vi "Script Find current Error Codes.vi"(8 "error in":errorcluster, 11 "Selection Owning Folder":path) -> (0 "error out":errorcluster, 1 "All Error VIS":path[](array[path]), 2 "Error and Descriptions Table":string[][](array[string]))   [LabVIEW 2020, in "ConstantErrorsMaker.lvlib"]
uses:
  ConstantErrorsMaker.lvlib
  <vilib>/Utility/traverseref.llb/TRef TravTarget.ctl
  c460e84f-7e8e-40e4-832a-a8e949bfd169.vi
  <vilib>/Comparison/Less/Less Functor/Less Functor.lvclass
  <vilib>/Utility/traverseref.llb/VI Scripting - Traverse.lvlib
  Error Info--cluster.ctl
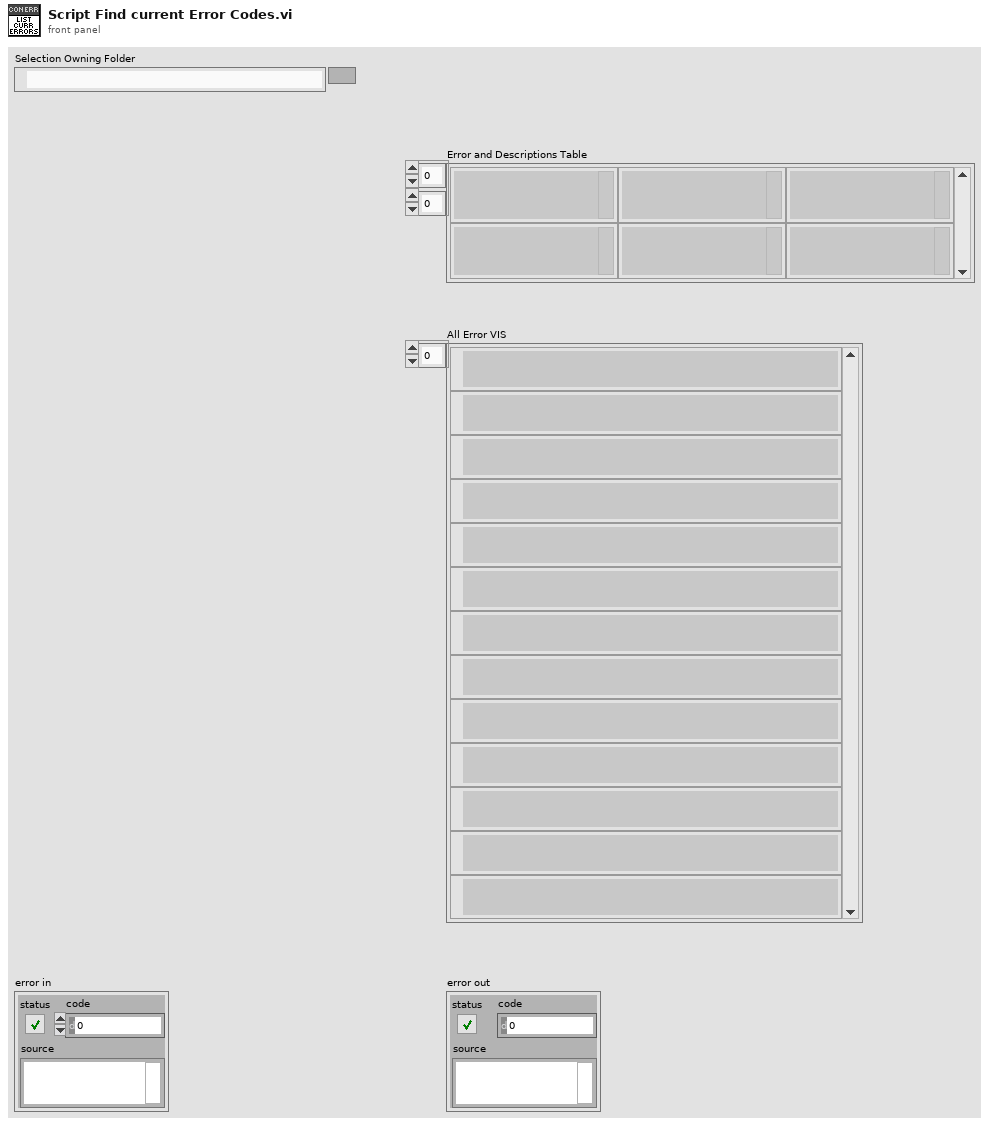
[diagram p1: front panel]
types:
  T1 = typedef "ConstantErrorsMaker.lvlib/Error Info--cluster.ctl" = cluster{"Error Code":i32, "Error Description":string, "Parent":string, "Error Path":path}
  T2 = typedef "TRef TravTarget.ctl" = enum16{"FP", "BD", "Other"}
  T3 = cluster{"Clipped Error Description":string, "Full Error Description":string, "code":i32, "Family":string, "Custom Description":string, "Is Error":bool, "Types":variant[], "Include Call Chain?":bool, "Error Text Visible":bool}
  T4 = cluster{"Library Version":cluster{"Major":u16, "Minor":u16, "Fix":u16, "Build":u16}, "State":variant}
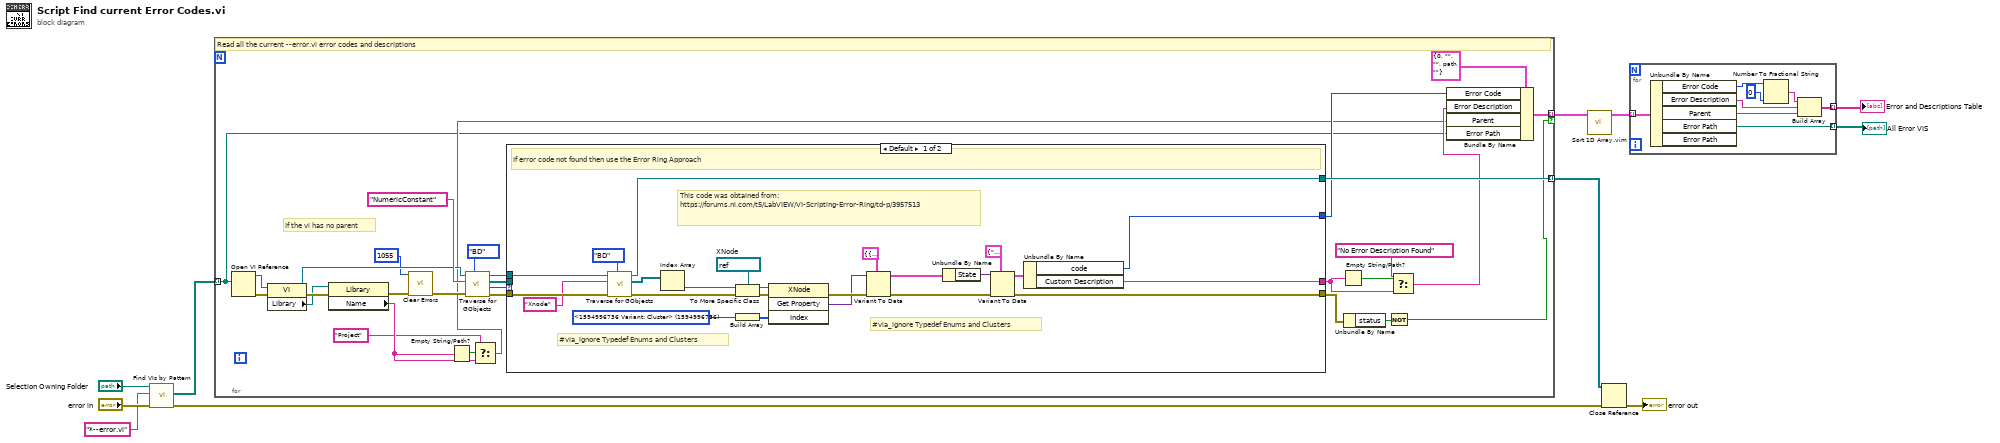
[diagram p0: block diagram]
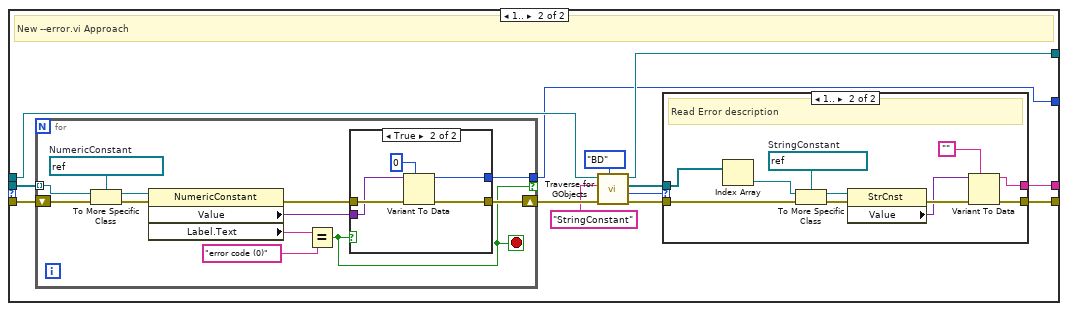
[diagram p2: hidden frame]
diagram:
  n1 = call "Find VIs by Pattern.vi"("error in"="error in", "pattern"="*--error.vi", "Selction Owning Folder"="Selection Owning Folder") -> ("error out"=w10:errorcluster, "All Files in Dir"=w7:path[])  [unwired: 7 in]
  n2 = for {
    tunnel: w7 -> [w12] mode=indexing
    tunnel: [w30] -> w6 mode=indexing
    tunnel: [w17] -> w4 mode=indexing if=w16
    # "If the vi has no parent"
    # "Read all the current --error.vi error codes and descriptions"
    n3 = Open VI Reference(vi path=w12) -> (vi reference=w25:refnum<vi>, error out=w40:errorcluster)  [unwired: 5 in]
    n4 = property class="VI"(reference=w25, error in=w40) -> (reference out=w24:refnum<vi>, error out=w38:errorcluster, "Library"=w23:refnum<vi>)
    n5 = property class="Library"(reference=w23, error in=w38) -> (error out=w37:errorcluster, "Name"=w21:string)  [unwired: 1 out]
    n6 = call <vilib>:"Clear Errors.vi"("error in (no error)"=w37, "specific error code to clear (0: all)"=1055) -> ("error out"=w36:errorcluster)  [unwired: 4 in, 1 out]
    n7 = Empty String/Path?(string/path=w21) -> (empty?=w22:bool)
    n8 = call <vilib>:"Traverse for GObjects.vi"("Traverse Target"=TRef_TravTarget."BD", "error in (no error)"=w36, "Class Name"="NumericConstant", "VI Refnum"=w24) -> ("error out"=w41:errorcluster, "# of Refs"=w32:i32, "References"=w34:refnum<vi>[], "dup VI Refnum"=w31:refnum<vi>)  [unwired: 4 in]
    n9 = Select(t="Project", s=w22, f=w21) -> (s? t:f=w13:string)
    n10 = case shown="Default" w32 {
      tunnel: [w44 w66] -> w15
      tunnel: [w62 w77] -> w39
      tunnel: w41 -> [w65 w76]
      tunnel: w34 -> [_ w74]
      tunnel: w31 -> [w57 w69]
      tunnel: [w43 w68] -> w27
      tunnel: [w42 w67] -> w30
      frame Default {
        w53 = u32 1594996736 items=["<1594996736 Variant: Cluster>"=1594996736, "<1594996767 Diagram RefNum>"=1594996737, "<1594996738 ProjectItem Refnum>"=1594996738, "<1594996739 Boolean>"=1594996739, "<1594996740 Boolean>"=1594996740, "<1594996741 Boolean>"=1594996741, "<1594996742 String: .html file name>"=1594996742, "<1594996743 Help Path>"=1594996743, "<1594996744 String: Tip Strip>"=1594996744, "<1594996745 Boolean>"=1594996745, "<104204298 Boolean>"=104204298, "AutoSize To Fit Contents?"=104204288, "Basic Object Flags"=103983116, "Bounds"=103983107, "Bounds:Area Height"=103983109, "Bounds:Area Width"=103983108, "Breakpoint Status"=104173580, "Clump Num"=104173572, "Content Rect"=104204293, "Description"=104173570, "Diagrams[]"=104204291, "Fire Count"=104173574, "Fix Contents"=104204297, "Frame Size"=104204290, "Icon"=104173576, "Is Asynchronous"=104173575, "Is Break Point Set"=104173571, "Is Run At Any Loop"=104173578, "Is Wizard Locked"=103983117, "Label"=104173569, "Master Bounds Rect"=103983115, "Position"=103983104, "Position:Left"=103983105, "Position:Top"=103983106, "Resize Info:Can Resize Horizontally"=103983119, "Resize Info:Can Resize Vertically"=103983120, "Resize Info:Include In Resize"=103983122, "Resize Info:Name in Resize Dialog"=103983121, "Selected"=103983113, "Shared Clones:Automatic Allocation Strategy Enabled"=104204295, "Shared Clones:Pre-Allocate"=104204296, "Short Count"=104173573, "Style"=104173577, "Target Syntax Checking"=104204292, "Terminals[]"=104173568, "Total Bounds Rect"=103983114, "Tunnels[]"=104204289, "UID"=103983123]
        w56 = refnum<vi> refnum  # XNode
        # "#via_ignore Typedef Enums and Clusters"
        # "#via_ignore Typedef Enums and Clusters"
        # "This code was obtained from:\nhttps://forums.ni.com/t5/LabVIEW/VI-Scripting-Error-Ring/td-p/3957513"
        # "If error code not found then use the Error Ring Approach"
        n11 = call <vilib>:"Traverse for GObjects.vi"("Traverse Target"=TRef_TravTarget."BD", "error in (no error)"=w65, "Class Name"="Xnode", "VI Refnum"=w57) -> ("error out"=w64:errorcluster, "References"=w55:refnum<vi>[], "dup VI Refnum"=w42:refnum<vi>)  [unwired: 4 in, 1 out]
        n12 = Index Array(array=w55) -> (element=w54:refnum<vi>)  [unwired: 1 in]
        n13 = To More Specific Class(target class=w56, reference=w54, error in=w64) -> (specific class reference=w52:refnum<vi>, error out=w63:errorcluster)
        n14 = Build Array(w53) -> (w51:u32[])
        n15 = invoke class="XNode" method="Get Property"(reference=w52, error in=w63, "Index"=w51) -> (error out=w61:errorcluster, "GetProperty"=w46:variant)  [unwired: 1 in, 2 out]
        n16 = Variant To Data(error in=w61, type=T4 {"Library Version"={"Major"=0, "Minor"=0, "Fix"=0, "Build"=0}, "State"=variant} ("output cluster"), Variant=w46) -> (data=w50:T4, error out=w60:errorcluster)
        n17 = Unbundle By Name(w50) -> ("State"=w48:variant)
        n18 = Variant To Data(error in=w60, type=T3 {"Clipped Error Description"="", "Full Error Description"="", "code"=0, "Family"="", "Custom Description"="", "Is Error"=TRUE, "Types"=[], "Include Call Chain?"=TRUE, "Error Text Visible"=TRUE} ("State"), Variant=w48) -> (data=w45:T3, error out=w62:errorcluster)
        n19 = Unbundle By Name(w45) -> ("code"=w44:i32, "Custom Description"=w43:string)
      }
      frame 1.. {
        # "New --error.vi Approach"
        n20 = for {
          tunnel: w74 -> [w86] mode=indexing
          tunnel: [w80] -> w66 if=w79
          shift-right: [w87] -> w75
          shift-left: w76 -> [w90]
          stop <- w79 stop-if-true
          w85 = refnum<vi> refnum  # NumericConstant
          n21 = To More Specific Class(target class=w85, reference=w86, error in=w90) -> (specific class reference=w84:refnum<vi>, error out=w89:errorcluster)
          n22 = property class="NumericConstant"(reference=w84, error in=w89) -> (error out=w88:errorcluster, "Value"=w81:variant, "Label.Text"=w83:string)  [unwired: 1 out]
          n23 = Equal?(x=w83, y="error code (0)") -> (x = y?=w79:bool)
          n24 = case shown="True" w79 {
            tunnel: w81 -> [_ w93]
            tunnel: w88 -> [w91 w96]
            tunnel: [w91 w95] -> w87
            tunnel: [_ w92] -> w80
            frame False {
            }
            frame True {
              n25 = Variant To Data(error in=w96, type=0, Variant=w93) -> (data=w92:i32, error out=w95:errorcluster)
            }
          }
        }
        n26 = call <vilib>:"Traverse for GObjects.vi"("Traverse Target"=TRef_TravTarget."BD", "error in (no error)"=w75, "Class Name"="StringConstant", "VI Refnum"=w69) -> ("error out"=w78:errorcluster, "# of Refs"=w70:i32, "References"=w73:refnum<vi>[], "dup VI Refnum"=w67:refnum<vi>)  [unwired: 4 in]
        n27 = case shown="1.." w70 {
          tunnel: [_ w104] -> w68
          tunnel: [w97 w108] -> w77
          tunnel: w78 -> [w97 w107]
          tunnel: w73 -> [_ w99]
          frame Default {
          }
          frame 1.. {
            w103 = refnum<vi> refnum  # StringConstant
            # "Read Error description"
            n28 = Index Array(array=w99) -> (element=w98:refnum<vi>)  [unwired: 1 in]
            n29 = To More Specific Class(target class=w103, reference=w98, error in=w107) -> (specific class reference=w102:refnum<vi>, error out=w106:errorcluster)
            n30 = property class="StrCnst"(reference=w102, error in=w106) -> (error out=w105:errorcluster, "Value"=w101:variant)  [unwired: 1 out]
            n31 = Variant To Data(error in=w105, type="", Variant=w101) -> (data=w104:string, error out=w108:errorcluster)
          }
        }
      }
    }
    n32 = Empty String/Path?(string/path=w27) -> (empty?=w28:bool)
    n33 = Unbundle By Name(w39) -> ("status"=w29:bool)
    n34 = Not(x=w29) -> (.not. x?=w16:bool)
    n35 = Select(t="No Error Description Found", s=w28, f=w27) -> (s? t:f=w14:string)
    n36 = Bundle By Name(cluster=T1 {"Error Code"=0, "Error Description"="", "Parent"="", "Error Path"=path ""} ("Error Info"), "Error Code"=w15, "Error Description"=w14, "Parent"=w13, "Error Path"=w12) -> (w17:T1)
  }
  n37 = call "Sort 1D Array.vim"("unsorted array"=w4) -> ("sorted array"=w3:T1[])  [unwired: 10 in]
  n38 = Close Reference(reference=w6, error in (no error)=w10) -> (error out=→"error out":errorcluster)
  n39 = for {
    tunnel: w3 -> [w116] mode=indexing
    tunnel: [w110] -> w1 mode=indexing
    tunnel: [w109] -> w2 mode=indexing
    n40 = Unbundle By Name(w116) -> ("Error Code"=w114:i32, "Error Description"=w112:string, "Parent"=w111:string, "Error Path"=w110:path)  [unwired: 1 out]
    n41 = Number To Fractional String(number=w114, precision (6)=i16 0) -> (F-format string=w113:string)  [unwired: 2 in]
    n42 = Build Array(w113, w112, w111) -> (w109:string[])
  }
  "Error and Descriptions Table" <- w2
  "All Error VIS" <- w1
